vi "xiCam - StopAcquisition.vi"(8 "error in (no error)":errorcluster, 11 "xiCam In":refnum<k24>) -> (0 "error out":errorcluster, 3 "xiCam Out":refnum<k24>)   [LabVIEW 2015]
doc: "This function stops the work cycle and data acquisition on the device.\n\n<b>void StopAcquisition()</b>"
uses:
  C:/GIT/Cameras3.x/Integrations/Labview/xiLib/xiLIB_32bit/xiLIB/xiCamLib/API/x86/xiApi.NET.dll
  xiLIB_32bit/xiLIB/xiCamLib/API/x86/xiApi.NET.dll
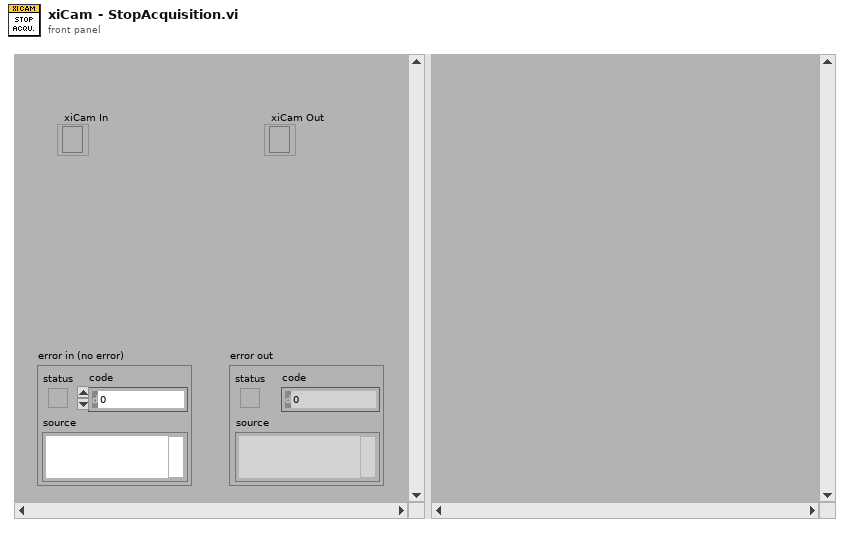
[diagram p1: front panel]
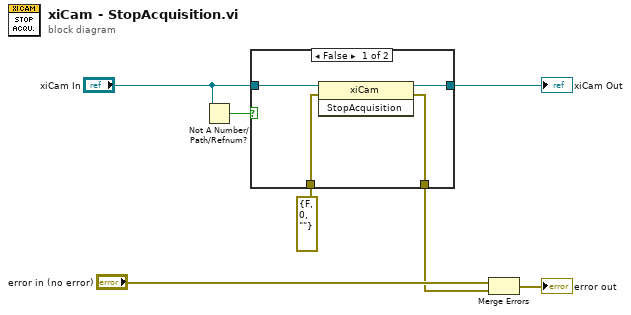
[diagram p0: block diagram]
diagram:
  n1 = Not A Number/Path/Refnum?(number/path/refnum="xiCam In") -> (NaN/Path/Refnum?=w5:bool)
  n2 = case shown="False" w5 {
    tunnel: [w11 w13] -> w6
    tunnel: errorcluster {"status"=FALSE, "code"=0, "source"=""} ("error in (no error) 2") -> [w10 w12]
    tunnel: [w9 w12] -> w2
    tunnel: "xiCam In" -> [w8 w13]
    frame False {
      n3 = invoke class="xiCam" method="StopAcquisition"(reference=w8, error in=w10) -> (reference out=w11:refnum<k24>, error out=w9:errorcluster)  [unwired: 1 in, 1 out]
    }
    frame True {
    }
  }
  "xiCam Out" <- w6
  n4 = Merge Errors("error in (no error)", w2) -> (→"error out":errorcluster)
